vi "Configure Heater Output 2 Advanced Operation.vi"(0 "VISA resource name":refnum<visa-resource-name>, 5 "Monitor Units (1:Kelvin)":u16(ring)=1 items=["Kelvin"=1, "Celsius"=2, "Sensor Units"=3], 7 "Monitor High Value (0.0000)":dbl format="%.4f", 9 "Monitor Low Value (0.0000)":dbl format="%.4f", 11 "error in (no error)":errorcluster, 12 "Control (0:Auto Off)":u16(ring) items=["Auto Off", "Continuous"], 13 "Percentage of Full Scale (0.00 %)":dbl format="%.2f") -> (4 "VISA resource name out":refnum<visa-resource-name>, 15 "error out":errorcluster)   [LabVIEW 2019, in "Lake Shore 335.lvlib"]
doc: "Configures the Monitor Output and Warmup Supply settings for heater output 2. \n\n<B>Use the Configure Heater Outputs VI to set the output 2 Mode to Monitor Out or Warmup Supply and Output Type to Voltage before using this VI.</B> \n\nIn Monitor Out mode, the voltage output (Output 2) tracks the assigned Control Input according to the scaling parameters you entered. Warm Up Supply mode is designed for controlling an external power supply used for rapidly increasing the temperature in the controlled system, for example, to bring a system to room temperature in order to change samples.\n\nWarm Up Supply mode is designed for controlling an external power supply used for rapidly increasing the temperature in the controlled system, for example, to bring a system to room temperature in order to change samples."
uses:
  Lake Shore 335.lvlib
panel:
  # "Monitor Output Settings (Mode = Monitor Out, Output Type = Voltage)"
  # "Warmup Supply Settings (Mode = Warmup Supply, Output Type = Voltage)"
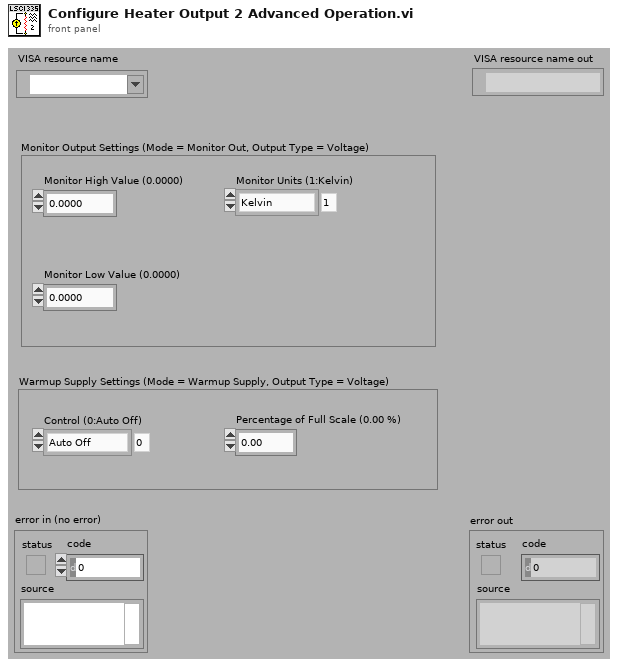
[diagram p1: front panel]
types:
  T1 = typedef "Lake Shore 335.lvlib/Extended User Data.ctl" = cluster{"Mode (0:Off)":u16, "Polarity (0:Unipolar)":u16, "Output Type (0:Current)":u16, "Input (0:None)":u16}
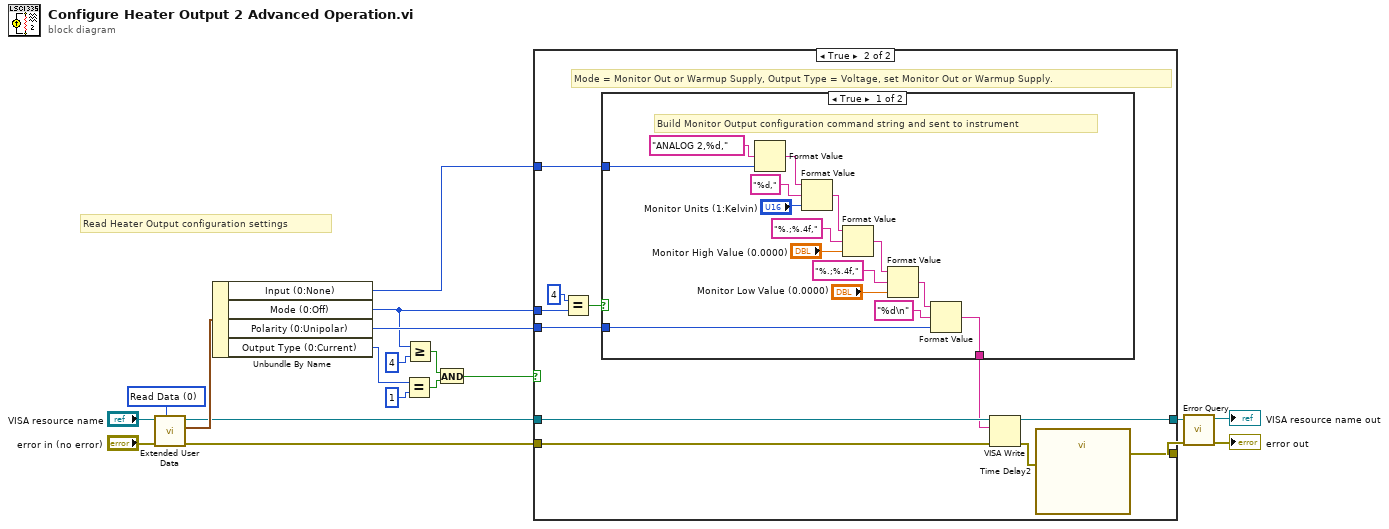
[diagram p0: block diagram]
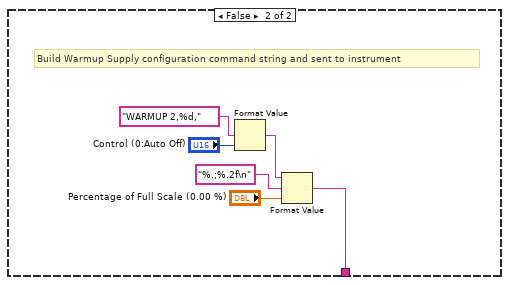
[diagram p3: hidden frame]
diagram:
  w15 = u16 0 items=["Read Data", "Write Data", "Clear Data", "Clear ALL Data"] ("Action")
  # "Read Heater Output configuration settings"
  n1 = call "Extended User Data.vi"("Action"=w15, "Error In (no error)"="error in (no error)", "VISA resource name in"="VISA resource name") -> ("Error Out"=w9:errorcluster, "User Data Out"=w14:T1, "VISA resource name out"=w10:refnum<visa-resource-name>)  [unwired: 6 in]
  n2 = Unbundle By Name(w14) -> ("Input (0:None)"=w1:u16, "Mode (0:Off)"=w6:u16, "Polarity (0:Unipolar)"=w11:u16, "Output Type (0:Current)"=w13:u16)
  n3 = Equal?(x=w13, y=u16 1) -> (x = y?=w4:bool)
  n4 = Greater Or Equal?(x=w6, y=u16 4) -> (x >= y?=w3:bool)
  n5 = And(x=w3, y=w4) -> (x .and. y?=w2:bool)
  n6 = case shown="True" w2 {
    tunnel: w6 -> [_ w24]
    tunnel: w11 -> [_ w32]
    tunnel: w10 -> [w21 w30]
    tunnel: w9 -> [w20 w29]
    tunnel: [w21 w28] -> w8
    tunnel: [w20 w27] -> w7
    tunnel: w1 -> [_ w22]
    frame False {
      # "Mode does not = Monitor Out or Warmup supply, or Output Type = Current.\nDo not set Monitor Out or Warmup Supply."
    }
    frame True {
      # "Mode = Monitor Out or Warmup Supply, Output Type = Voltage, set Monitor Out or Warmup Supply."
      n7 = Equal?(x=u16 4, y=w24) -> (x = y?=w25:bool)
      n8 = case shown="True" w25 {
        tunnel: w32 -> [w35 _]
        tunnel: [w34 w48] -> w26
        tunnel: w22 -> [w33 _]
        frame True {
          # "Build Monitor Output configuration command string and sent to instrument"
          n9 = Format Value(format string="ANALOG 2,%d,", value (0)=w33) -> (output string=w44:string)  [unwired: 1 in]
          n10 = Format Value(string ("")=w44, format string="%d,", value (0)="Monitor Units (1:Kelvin)") -> (output string=w42:string)
          n11 = Format Value(string ("")=w42, format string="%.;%.4f,", value (0)="Monitor High Value (0.0000)") -> (output string=w41:string)
          n12 = Format Value(string ("")=w41, format string="%.;%.4f,", value (0)="Monitor Low Value (0.0000)") -> (output string=w40:string)
          n13 = Format Value(string ("")=w40, format string="%d\n", value (0)=w35) -> (output string=w34:string)
        }
        frame False {
          # "Build Warmup Supply configuration command string and sent to instrument"
          n14 = Format Value(format string="WARMUP 2,%d,", value (0)="Control (0:Auto Off)") -> (output string=w52:string)  [unwired: 1 in]
          n15 = Format Value(string ("")=w52, format string="%.;%.2f\n", value (0)="Percentage of Full Scale (0.00 %)") -> (output string=w48:string)
        }
      }
      n16 = VISA Write(VISA resource name=w30, write buffer=w26, error in (no error)=w29) -> (VISA resource name out=w28:refnum<visa-resource-name>, error out=w31:errorcluster)  [unwired: 1 out]
      n17 = call "Time Delay2"("error in (no error)"=w31) -> ("error out"=w27:errorcluster)  [unwired: 10 in]
    }
  }
  n18 = call "Error Query.vi"("error in (no error)"=w7, "VISA resource name"=w8) -> ("error out"=→"error out":errorcluster, "VISA resource name out"=→"VISA resource name out":refnum<visa-resource-name>)  [unwired: 7 in, 1 out]
